vi "ParseSortSplit.vi"(5 "AE Groups":T1[](array[typedef])=[enum."AE-Germany", enum."AE-Poland", enum."AE-Switzerland", enum."AE-Czech Republic", enum."AE-Hungary", enum."AE-Romania", enum."AE-Slovakia", enum."AE-Slovenia"], 6 "Older SRs on top?":bool, 7 "AE/ELP?":bool, 8 "Error In":errorcluster, 11 "SR List In":T2[](array[typedef])) -> (0 "Error Out":errorcluster, 2 "Unassigned SR List":T2[](array[typedef]), 3 "Assigned SR List":T2[](array[typedef]))   [LabVIEW 2017, in "Client.lvlib"]
uses:
  Client.lvlib
  ParserSorter/TypeDefs/SRData.ctl
  ParserSorter/TypeDefs/AEGroup.ctl
  ParserSorter/TypeDefs/SRStatus.ctl
  ParserSorter/TypeDefs/SRLevel.ctl
  ParserSorter/TypeDefs/SRType.ctl
  ParserSorter/ParserSorter.lvlib
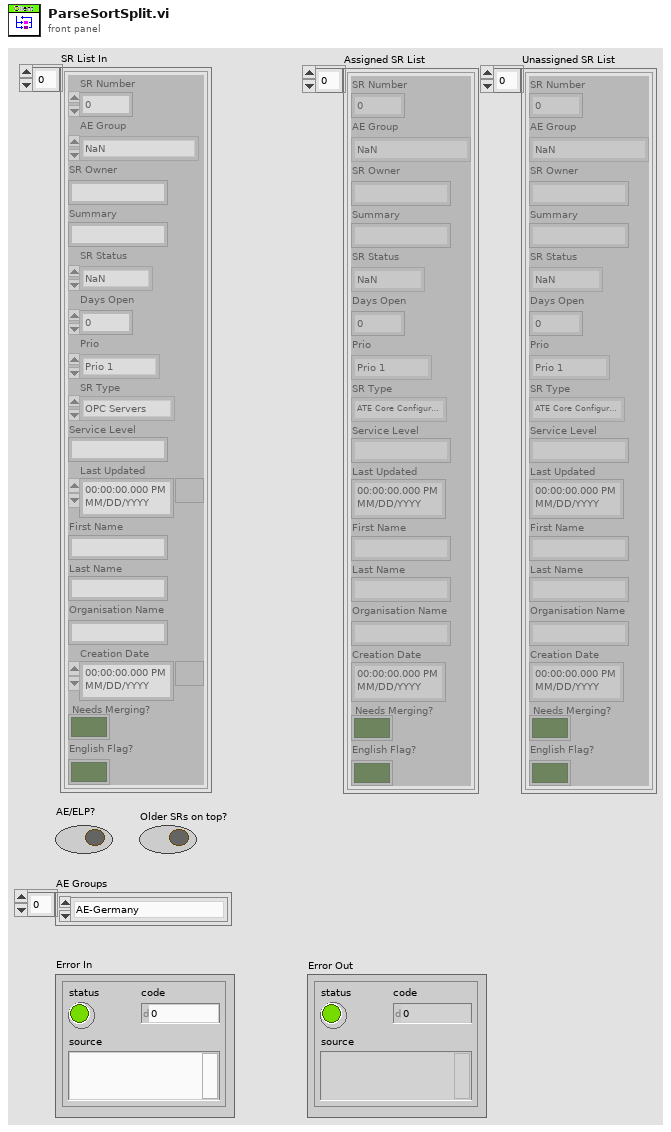
[diagram p1: front panel]
types:
  T1 = typedef "Client.lvlib/ParserSorter.lvlib/AEGroup.ctl" = enum32{"NaN", "AE-Germany", "AE-Poland", "AE-Switzerland", "AE-Czech Republic", "AE-Hungary", "AE-Romania", "AE-Slovakia", "AE-Slovenia"}
  T2 = typedef "Client.lvlib/ParserSorter.lvlib/SRData.ctl" = cluster{"SR Number":i64, "AE Group":T1, "SR Owner":string, "Summary":string, "SR Status":T3, "Days Open":dbl, "Prio":T4, "SR Type":T5, "Service Level":string, "Last Updated":timestamp, "First Name":string, "Last Name":string, "Organisation Name":string, "Creation Date":timestamp, "Needs Merging?":bool, "English Flag?":bool}
  T3 = typedef "Client.lvlib/ParserSorter.lvlib/SRStatus.ctl" = enum32{"NaN", "Caller Abandoned", "Created in Error", "Declined to Purchase Support", "Expired", "Forum Resolved AE", "Forum Resolved Customer", "IN WORK", "IN WORK Collab with AES", "IN WORK Collab with PSE", "IN WORK Collab with SE", "IN WORK Escalation", "IN WORK Customer Added Note", "Open", "Potentially Resolved", "POC Resolved", "Resolved", "RMA Waiting on Customer", "RMA Open", "RMA In Progress", "RMA Closed - DOA", "RMA Closed", "RMA Approved for Return", "Project Complete", "Presumed Resolved", "IN WORK Wait on Customer"}
  T4 = typedef "Client.lvlib/ParserSorter.lvlib/SRLevel.ctl" = enum16{"Prio 1", "Prio 2", "Prio 3", "Prio 4"}
  T5 = typedef "Client.lvlib/ParserSorter.lvlib/SRType.ctl" = enum32{"NaN", "ATE Core Configurations (BYOATE)", "Activation", "BioBench", "CAN", "CM C Series", "Calibration", "Consulting Services", "CounterTimer", "DAQExpress", "DASYLab", "DIAdem", "DMM", "DSA HW", "Digital_IO", "FIRST (NIC Only)", "FieldBus", "FieldPoint", "Functional Savety", "GATI", "GPIB", "HMI and Industrial PCs", "HiQ", "HighSpeedDigital_IO", "IMAQ", "IOTech Vibration", "Industrial Communications", "InsightCM", "LV", "LV CD&Sim", "LV Comms", "LV Controls Add-Ons", "LV Embedded", "LV MathScript RT", "LV NXG", "LV NXT", "LVDSC", "LVFPGA", "LVPDA and LV Touch Panel", "LVRT", "LabWindows_CVI", "Lookout", "MATRIXx", "MStudioDotNet", "MStudioVisualBasic", "MStudioVisualC", "Measure (Legacy)", "Motion", "MultifunctionDAQ", "Multimedia Test HW/SW", "Multisim (EWB)", "NI Update Service", "OPC Servers", "Optical (OSI)", "PXI Controllers, Chassis, MXI", "PXI Timing and Sync", "Power Supplies and SMUs", "Powertrain Controls", "RAID", "RF", "RF Software", "RIO", "SC Express", "SCC", "SCXI", "SPEEDY-33 (Hyperception)", "STS", "ScopeDigitizers", "Serial", "Signal Sources", "SignalCondOther", "SignalExpress", "Software Defined Intruments", "Sound and Vibration SW", "Switch Executive", "Switches", "TestStand", "USRP", "Ultiboard (EWB)", "VBench", "VI Logger", "VXI_MXI", "VeriStand", "VisionSW", "VolumeLicenseMgr", "WSN", "Web UI Builder", "myRIO"}
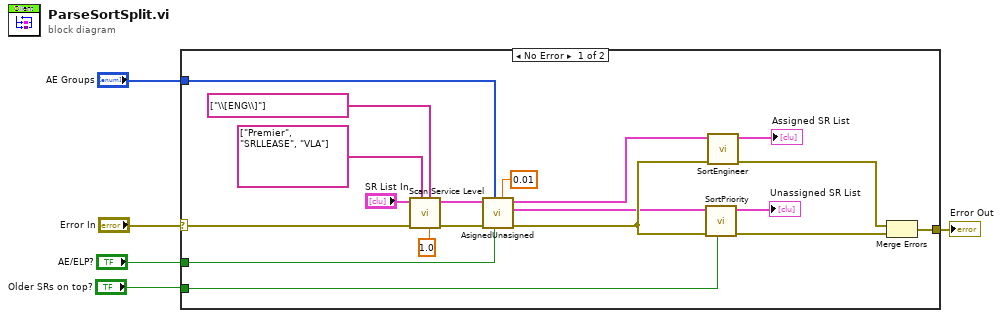
[diagram p0: block diagram]
diagram:
  n1 = case shown="No Error" "Error In" {
    selector: "Error In" -> [w21 w25]
    tunnel: [w13 w25] -> w4
    tunnel: "AE Groups" -> [w8 _]
    tunnel: "AE/ELP?" -> [w7 _]
    tunnel: "Older SRs on top?" -> [w6 _]
    frame No Error {
      n2 = call "Scan Service Level.vi"("Days Open Prio Threshold"=1.0, "English Tags"=string[] ["\\[ENG\\]"], "Premier Levels Keywords"=string[] ["Premier", "SRLLEASE", "VLA"], "error in (no error)"=w21, "Array in"="SR List In") -> ("error out"=w20:errorcluster, "Array out"=w19:T2[])  [unwired: 5 in]
      n3 = call "AsignedUnasigned.vi"("Days Open Phone Treshhold"=0.01, "AE/ELP?"=w7, "AE Groups"=w8, "error in (no error)"=w20, "All SR In"=w19) -> ("error out"=w17:errorcluster, "Unassigned"=w15:T2[], "Assigned Out"=w16:T2[])  [unwired: 4 in]
      n4 = call "SortPriority.vi"("Older SRs on top?"=w6, "error in (no error)"=w17, "Array in"=w15) -> ("error out"=w11:errorcluster, "Array out"=→"Unassigned SR List":T2[])  [unwired: 7 in]
      n5 = call "SortEngineer.vi"("error in (no error)"=w17, "Array in"=w16) -> ("error out"=w12:errorcluster, "Array out"=→"Assigned SR List":T2[])  [unwired: 8 in]
      n6 = Merge Errors(w12, w11) -> (w13:errorcluster)
    }
    frame Error {
    }
  }
  "Error Out" <- w4
